vi "Elevator_Execute.vi"() -> ()   [LabVIEW 2019]
uses:
  Climb_Globals.vi
  <vilib>/Rock Robotics/WPI/ThirdParty/Phoenix-LabVIEW/Motor Controller/Controls/CTRE_Phoenix_MotorControl_ControlMode.ctl
  Globals/Sensor_Values.vi
  Globals/Solenoid Globals.vi
  <vilib>/Rock Robotics/WPI/Solenoid/WPI_SolenoidValue.ctl
  <vilib>/Rock Robotics/WPI/Solenoid/WPI_SolenoidSetEnum.vi
panel:
  in  "BrakeDelay(ms)":u32
  in  "acceptable_error":dbl
  out "Waveform Chart":dbl(graph)=252.0
  out "Left_Value_Added":dbl
  out "Right_Value_Added":dbl
  out "difference(left-right)":dbl=252.0
  out "Left_Side_Input":dbl
  out "Right_Side_Input":dbl
  in  "Left Down %V P-Gain":dbl=0.0003
  in  "Right Down %V P-Gain":dbl=0.0003
  in  "Left SpeedControl P-Gain":dbl
  in  "Right SpeedControl P-Gain":dbl
  in  "Max_Elevator_Speed":dbl
  in  "Left Up %V P-Gain":dbl=0.0003
  in  "Right Up %V P-Gain":dbl=0.0003
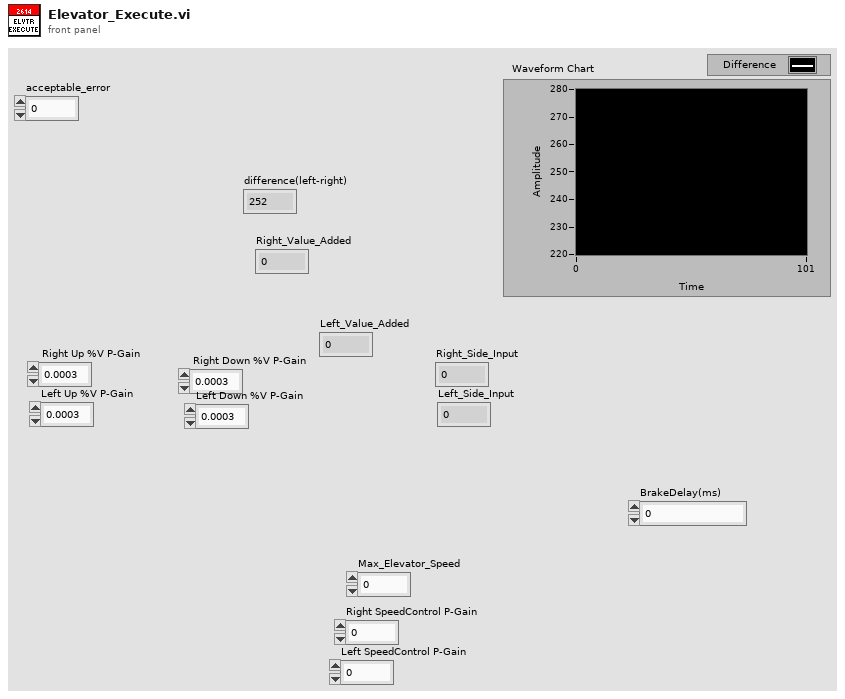
[diagram p1: front panel]
types:
  T1 = typedef "WPI_MotorControlDeviceRef.ctl" = cluster{"DeviceStatus":errorcluster, "Type":T2, "PWM":cluster{"PWM Channel":T3, "DeadBand":T4}, "CAN":cluster{"Device Number":u8, "SetOutput VI Ref":variant, "GetOutput VI Ref":variant, "Enable VI Ref":variant, "Disable VI Ref":variant, "Data":variant}, "Invert":bool, "DIO PWM":cluster{"PWM \"Enable\" Channel":T3, "DIOChannel":T5, "PWM Rate":dbl}}
  T2 = typedef "WPI_MotorControlType.ctl" = enum16{"PWM", "CAN", "DIO PWM"}
  T3 = typedef "FPGA_DIOPWMChannel.ctl" = enum8{"PWM 0", "PWM 1", "PWM 2", "PWM 3", "PWM 4", "PWM 5", "PWM 6", "PWM 7", "PWM 8", "PWM 9", "PWM MXP 0", "PWM MXP 1", "PWM MXP 2", "PWM MXP 3", "PWM MXP 4", "PWM MXP 5", "PWM MXP 6", "PWM MXP 7", "PWM MXP 8", "PWM MXP 9", "Invalid"}
  T4 = typedef "WPI_PWMDeadband.ctl" = cluster{"Name":string, "maxPositivePwm":i32, "minPositivePwm":i32, "centerPwm":i32, "maxNegativePwm":i32, "minNegativePwm":i32, "angularRange":u16}
  T5 = typedef "FPGA_DIOChannel.ctl" = enum8{"DIO 0", "DIO 1", "DIO 2", "DIO 3", "DIO 4", "DIO 5", "DIO 6", "DIO 7", "DIO 8", "DIO 9", "DIO MXP 0", "DIO MXP 1", "DIO MXP 2", "DIO MXP 3", "DIO MXP 4", "DIO MXP 5", "DIO MXP 6", "DIO MXP 7", "DIO MXP 8", "DIO MXP 9", "DIO MXP 10", "DIO MXP 11", "DIO MXP 12", "DIO MXP 13", "DIO MXP 14", "DIO MXP 15", "SPI Port CS1", "SPI Port CS2", "SPI Port CS3", "SPI Port MISO", "SPI Port MOSI", "Invalid"}
  T6 = typedef "WPI_SolenoidDevRef.ctl" = cluster{"DevStatus":errorcluster, "Pneumatics Control Module":u8, "Forward Solenoid Channel":T7, "Reverse Solenoid Channel":T7}
  T7 = typedef "WPI_SolenoidChannel.ctl" = enum8{"Solenoid 0", "Solenoid 1", "Solenoid 2", "Solenoid 3", "Solenoid 4", "Solenoid 5", "Solenoid 6", "Solenoid 7", "Invalid"}
  T8 = typedef "WPI_SolenoidValue.ctl" = enum16{"Off", "On", "Forward", "Reverse"}
  T9 = typedef "Climb_Elevator_Cluster.ctl" = cluster{"Extend?":bool, "Elevator_Throttle":dbl, "Control_States":T10}
  T10 = typedef "Climb_Elevator_Control_States.ctl" = enum16{"No-Op", "Brake", "Going_Up", "Going_Down", "Manual_PercentVoltage", "Manual_SpeedControl"}
  T11 = typedef "CTRE_Phoenix_MotorControl_ControlMode.ctl" = u16
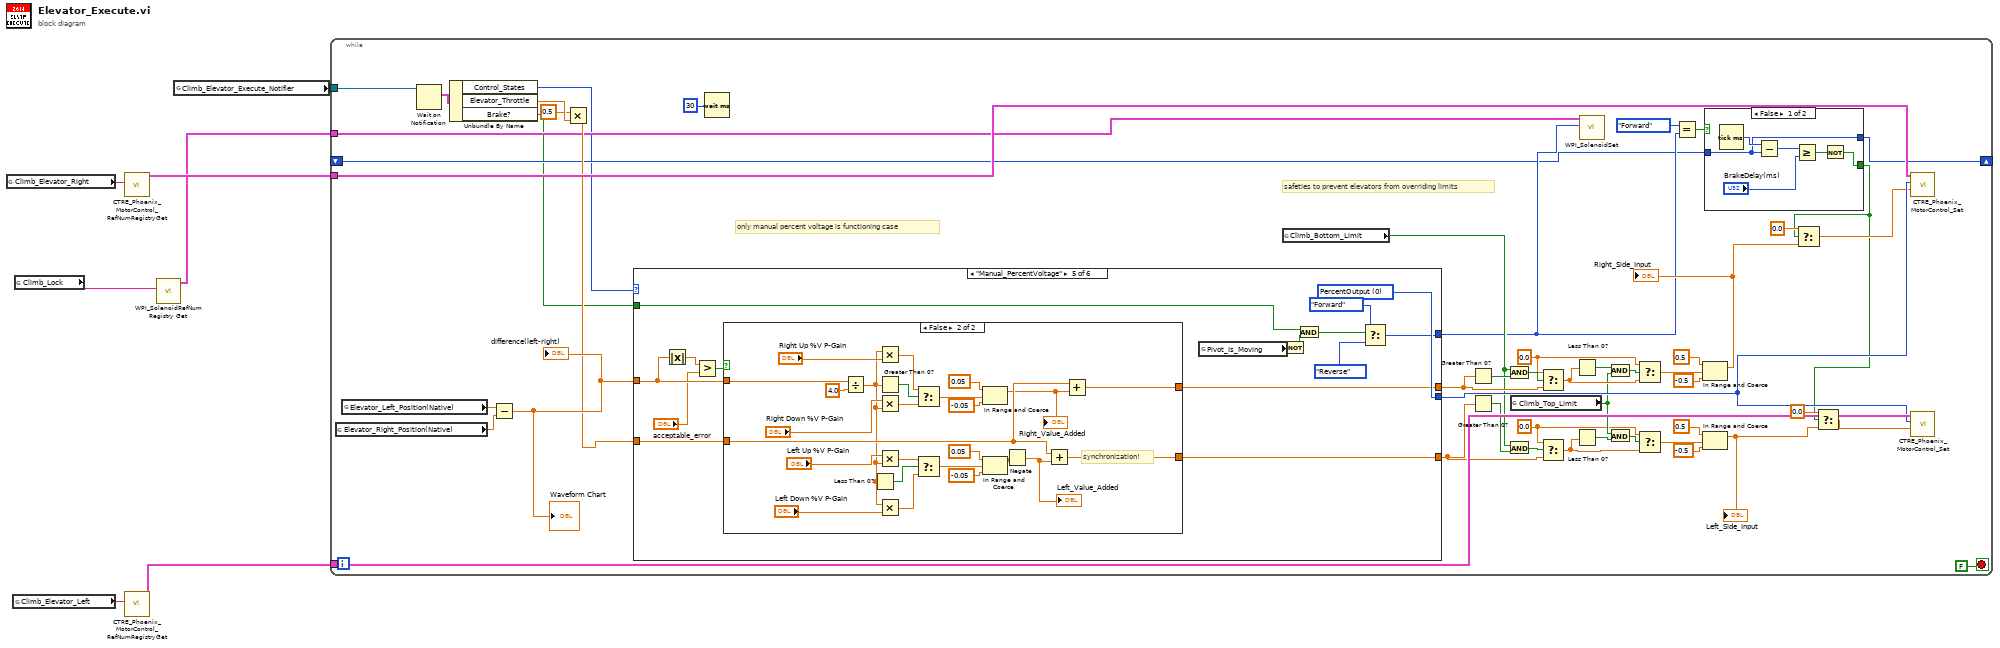
[diagram p0: block diagram]
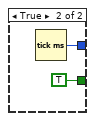
[diagram p2: hidden frame]
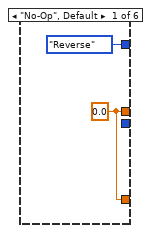
[diagram p3: hidden frame]
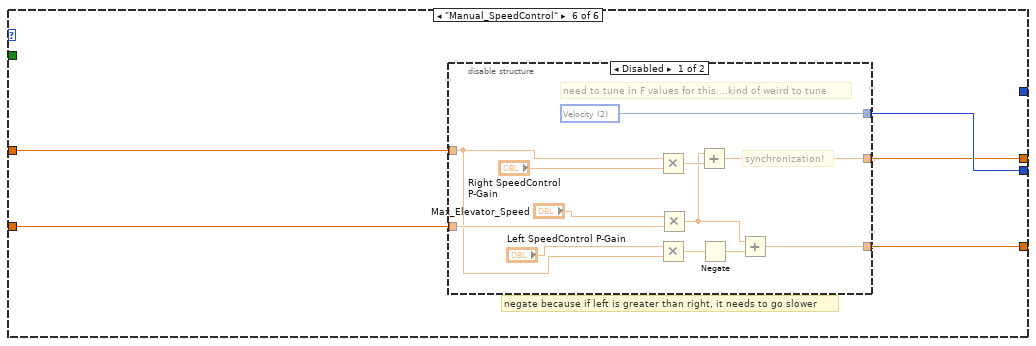
[diagram p8: hidden frame]
diagram:
  n1 = global read "Climb_Globals.vi" "Climb_Elevator_Right"() -> (w4:string)
  n2 = global read "Climb_Globals.vi" "Climb_Elevator_Left"() -> (w3:string)
  n3 = global read "Solenoid Globals.vi" "Climb_Lock"() -> (w2:string)
  n4 = call <vilib>:"CTRE_Phoenix_MotorControl_RefNumRegistryGet.vi"("refnum name"=w4) -> ("PhoenixMotorControlDevRef"=w6:T1)  [unwired: 9 in, 1 out]
  n5 = call <vilib>:"CTRE_Phoenix_MotorControl_RefNumRegistryGet.vi"("refnum name"=w3) -> ("PhoenixMotorControlDevRef"=w5:T1)  [unwired: 9 in, 1 out]
  n6 = call <vilib>:"WPI_SolenoidRefNum Registry Get.vi"("refnum name"=w2) -> ("SolenoidDevRef"=w1:T6)  [unwired: 9 in, 1 out]
  n7 = global read "Climb_Globals.vi" "Climb_Elevator_Execute_Notifier"() -> (w7:refnum<notifier>)
  n8 = while {
    tunnel: w7 -> [w56]
    tunnel: w6 -> [w54]
    tunnel: w5 -> [w55]
    tunnel: w1 -> [w22]
    shift-right: [w11] -> _
    shift-left: _ -> [w10]
    stop <- FALSE stop-if-true
    w38 = 0.0 ("t")
    w42 = 0.0 ("t")
    # "only manual percent voltage is functioning case"
    # "safeties to prevent elevators from overriding limits"
    n9 = global read "Sensor_Values.vi" "Elevator_Right_Position(Native)"() -> (w52:dbl)
    n10 = global read "Sensor_Values.vi" "Elevator_Left_Position(Native)"() -> (w51:dbl)
    n11 = Wait on Notification(notifier=w56) -> (notification=w26:T9)  [unwired: 3 in, 3 out]
    n12 = Unbundle By Name(w26) -> ("Control_States"=w9:T10, "Elevator_Throttle"=w25:dbl, "Brake?"=w8:bool)
    n13 = Subtract(x=w51, y=w52) -> (x-y=w27:dbl)
    "difference(left-right)" <- w27
    "Waveform Chart" <- w27
    n14 = Multiply(x=0.5, y=w25) -> (x*y=w24:dbl)
    n15 = case shown="\"Manual_PercentVoltage\"" w9 {
      tunnel: w24 -> [_ _ _ _ w73 w112]
      tunnel: [_ _ _ _ w82 w113] -> w53
      tunnel: w27 -> [_ _ _ _ w79 w111]
      tunnel: [w67 _ _ _ w80 w109] -> w48
      tunnel: [w67 _ _ _ w81 w110] -> w30
      tunnel: [WPI_SolenoidValue."Reverse" ("Value") _ _ _ w75 _] -> w17
      tunnel: w8 -> [_ _ _ _ w70 _]
      frame "No-Op", Default {
        w67 = 0.0
      }
      frame "Brake" {
      }
      frame "Going_Up" {
      }
      frame "Going_Down" {
      }
      frame "Manual_PercentVoltage" {
        w82 = T11 0 items=["PercentOutput"=0, "Position"=1, "Velocity"=2, "Current"=3, "Follower"=5, "MotionProfile"=6, "MotionMagic"=7, "MotionProfileArc"=10, "Disabled"=15] ("Control Mode")
        n16 = Absolute Value(x=w79) -> (abs(x)=w77:dbl)
        n17 = Greater?(x=w77, y="acceptable_error") -> (0:w78:bool)
        n18 = case shown="False" w78 {
          tunnel: w73 -> [w83 w107]
          tunnel: [w83 w105] -> w80
          tunnel: [w83 w104] -> w81
          tunnel: w79 -> [_ w97]
          frame True {
          }
          frame False {
            # "synchronization!"
            n19 = Divide(x=w97, y=4.0) -> (x/y=w84:dbl)
            n20 = Less Than 0?(x=w84) -> (x < 0?=w85:bool)
            n21 = Multiply(x=w84, y="Right Up %V P-Gain") -> (x*y=w92:dbl)
            n22 = Multiply(x="Right Down %V P-Gain", y=w84) -> (x*y=w91:dbl)
            n23 = Multiply(x="Left Up %V P-Gain", y=w84) -> (x*y=w88:dbl)
            n24 = Multiply(x=w84, y="Left Down %V P-Gain") -> (x*y=w87:dbl)
            n25 = Greater Than 0?(x=w84) -> (x > 0?=w93:bool)
            n26 = Select(t=w92, s=w93, f=w91) -> (s? t:f=w90:dbl)
            n27 = Select(t=w88, s=w85, f=w87) -> (s? t:f=w86:dbl)
            n28 = In Range and Coerce(upper limit=0.05, x=w90, lower limit=-0.05) -> (coerced(x)=w98:dbl)  [unwired: 1 out]
            "Right_Value_Added" <- w98
            n29 = In Range and Coerce(upper limit=0.05, x=w86, lower limit=-0.05) -> (coerced(x)=w100:dbl)  [unwired: 1 out]
            n30 = Negate(x=w100) -> (-x=w103:dbl)
            "Left_Value_Added" <- w103
            n31 = Add(x=w107, y=w103) -> (x+y=w104:dbl)
            n32 = Add(x=w107, y=w98) -> (x+y=w105:dbl)
          }
        }
        n33 = global read "Climb_Globals.vi" "Pivot_Is_Moving"() -> (w69:bool)
        n34 = Not(x=w69) -> (.not. x?=w68:bool)
        n35 = And(x=w70, y=w68) -> (x .and. y?=w71:bool)
        n36 = Select(t=WPI_SolenoidValue."Forward" ("Value"), s=w71, f=WPI_SolenoidValue."Reverse" ("Value")) -> (s? t:f=w75:T8)
      }
      frame "Manual_SpeedControl" {
        # "negate because if left is greater than right, it needs to go slower"
        n37 = disable-structure shown="Disabled" {
          disable-tunnel: [w125 _] -> w113
          disable-tunnel: w112 -> [w124 _]
          disable-tunnel: w111 -> [w119 _]
          disable-tunnel: [w118 _] -> w110
          disable-tunnel: [w117 _] -> w109
          frame Disabled {
            w125 = T11 2 items=["PercentOutput"=0, "Position"=1, "Velocity"=2, "Current"=3, "Follower"=5, "MotionProfile"=6, "MotionMagic"=7, "MotionProfileArc"=10, "Disabled"=15] ("Control Mode")
            # "synchronization!"
            # "need to tune in F values for this....kind of weird to tune"
            n38 = Multiply(x=w119, y="Right SpeedControl P-Gain") -> (x*y=w122:dbl)
            n39 = Multiply(x="Left SpeedControl P-Gain", y=w119) -> (x*y=w121:dbl)
            n40 = Multiply(x="Max_Elevator_Speed", y=w124) -> (x*y=w116:dbl)
            n41 = Add(x=w116, y=w122) -> (x+y=w117:dbl)
            n42 = Negate(x=w121) -> (-x=w120:dbl)
            n43 = Add(x=w116, y=w120) -> (x+y=w118:dbl)
          }
          frame Enabled {
          }
        }
      }
    }
    n44 = Wait (ms)(milliseconds to wait=u32 30) -> ()  [unwired: 1 out]
    n45 = global read "Sensor_Values.vi" "Climb_Bottom_Limit"() -> (w46:bool)
    n46 = Greater Than 0?(x=w48) -> (x > 0?=w50:bool)
    n47 = Greater Than 0?(x=w30) -> (x > 0?=w29:bool)
    n48 = And(x=w46, y=w50) -> (x .and. y?=w49:bool)
    n49 = And(x=w46, y=w29) -> (x .and. y?=w47:bool)
    n50 = global read "Sensor_Values.vi" "Climb_Top_Limit"() -> (w40:bool)
    n51 = Select(t=w42, s=w49, f=w48) -> (s? t:f=w43:dbl)
    n52 = Select(t=w38, s=w47, f=w30) -> (s? t:f=w37:dbl)
    n53 = Less Than 0?(x=w43) -> (x < 0?=w44:bool)
    n54 = Less Than 0?(x=w37) -> (x < 0?=w39:bool)
    n55 = call-poly <vilib>:"WPI_SolenoidSet.vi"("Value"=w17, "SolenoidDevRef"=w22) -> ()  [unwired: 8 in, 2 out]
    n56 = And(x=w44, y=w40) -> (x .and. y?=w45:bool)
    n57 = And(x=w40, y=w39) -> (x .and. y?=w41:bool)
    n58 = Select(t=w42, s=w45, f=w43) -> (s? t:f=w31:dbl)
    n59 = Select(t=w38, s=w41, f=w37) -> (s? t:f=w36:dbl)
    n60 = Equal?(x=WPI_SolenoidValue."Forward", y=w17) -> (x = y?=w13:bool)
    n61 = In Range and Coerce(upper limit=0.5, x=w31, lower limit=-0.5) -> (coerced(x)=w21:dbl)  [unwired: 1 out]
    "Right_Side_Input" <- w21
    n62 = In Range and Coerce(upper limit=0.5, x=w36, lower limit=-0.5) -> (coerced(x)=w19:dbl)  [unwired: 1 out]
    "Left_Side_Input" <- w19
    n63 = case shown="False" w13 {
      tunnel: [w58 TRUE] -> w12
      tunnel: [w62 w64] -> w11
      tunnel: w10 -> [w62 _]
      frame False {
        n64 = Tick Count (ms)() -> (millisecond timer value=w63:u32)
        n65 = Subtract(x=w63, y=w62) -> (x-y=w61:u32)
        n66 = Greater Or Equal?(x=w61, y="BrakeDelay(ms)") -> (x >= y?=w59:bool)
        n67 = Not(x=w59) -> (.not. x?=w58:bool)
      }
      frame True {
        n68 = Tick Count (ms)() -> (millisecond timer value=w64:u32)
      }
    }
    n69 = Select(t=0.0, s=w12, f=w21) -> (s? t:f=w20:dbl)
    n70 = Select(t=0.0, s=w12, f=w19) -> (s? t:f=w18:dbl)
    n71 = call <vilib>:"CTRE_Phoenix_MotorControl_Set.vi"("Output"=w20, "Control Mode"=w53, "PhoenixMotorControlDevRef"=w54) -> ()  [unwired: 7 in, 2 out]
    n72 = call <vilib>:"CTRE_Phoenix_MotorControl_Set.vi"("Output"=w18, "Control Mode"=w53, "PhoenixMotorControlDevRef"=w55) -> ()  [unwired: 7 in, 2 out]
  }
